vi "DataRootifier.vi"(4 "pathPlaceholder":string, 6 "replacePathPortion":string, 8 "mode":enum16{"Generalise", "Localise"}(ring)=enum."Localise", 11 "pathIn":path) -> (3 "pathOut":path)   [LabVIEW 2022 SP3]
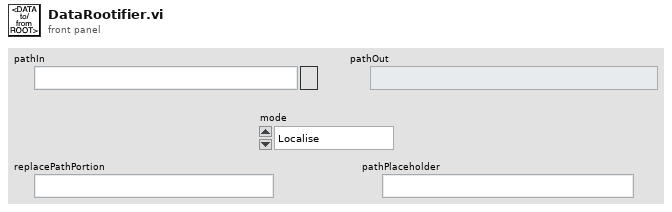
[diagram p1: front panel]
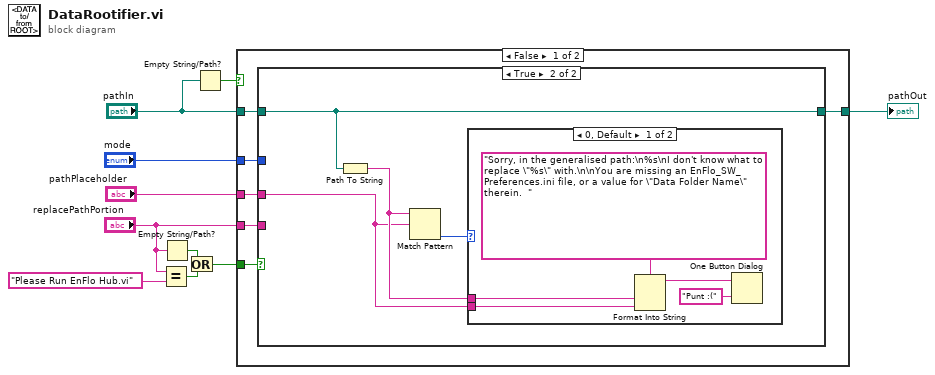
[diagram p0: block diagram]
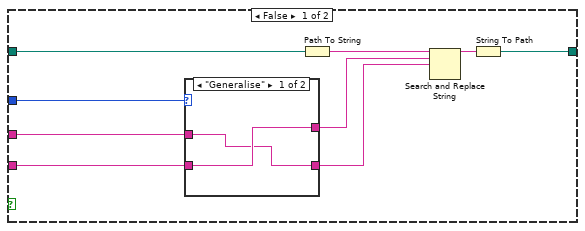
[diagram p2: hidden frame]
diagram:
  n1 = Equal?(x="replacePathPortion", y="Please Run EnFlo Hub.vi") -> (x = y?=w5:bool)
  n2 = Empty String/Path?(string/path="replacePathPortion") -> (empty?=w6:bool)
  n3 = Or(x=w6, y=w5) -> (x .or. y?=w7:bool)
  n4 = Empty String/Path?(string/path="pathIn") -> (empty?=w3:bool)
  n5 = case shown="False" w3 {
    tunnel: [w16 w39] -> w10
    tunnel: "pathIn" -> [w15 w39]
    tunnel: "replacePathPortion" -> [w14 _]
    tunnel: w7 -> [w13 _]
    tunnel: "pathPlaceholder" -> [w12 _]
    tunnel: "mode" -> [w11 _]
    frame False {
      n6 = case shown="True" w13 {
        tunnel: [w25 w33] -> w16
        tunnel: w15 -> [w22 w33]
        tunnel: w14 -> [w19 _]
        tunnel: w12 -> [w18 w30]
        tunnel: w11 -> [w17 _]
        frame False {
          n7 = case shown="\"Generalise\"" w17 {
            tunnel: [w27 w29] -> w21
            tunnel: w18 -> [w26 w29]
            tunnel: [w26 w28] -> w20
            tunnel: w19 -> [w27 w28]
            frame "Generalise" {
            }
            frame "Localise", Default {
            }
          }
          n8 = Path To String(path=w22) -> (string=w23:string)
          n9 = Search and Replace String(input string=w23, search string=w21, replace string=w20) -> (result string=w24:string)  [unwired: 5 in, 3 out]
          n10 = String To Path(string=w24) -> (path=w25:path)
        }
        frame True {
          n11 = Path To String(path=w33) -> (string=w31:string)
          n12 = Match Pattern(string=w31, regular expression=w30) -> (offset past match=w32:i32)  [unwired: 1 in, 3 out]
          n13 = case shown="0, Default" w32 {
            tunnel: w31 -> [w38 _]
            tunnel: w30 -> [w37 _]
            frame 0, Default {
              n14 = Format Into String(format string="Sorry, in the generalised path:\n%s\nI don't know what to replace \"%s\" with.\n\nYou are missing an EnFlo_SW_Preferences.ini file, or a value for \"Data Folder Name\" therein.  ", w38, w37) -> (resulting string=w35:string)  [unwired: 2 in, 1 out]
              n15 = One Button Dialog(message=w35, button name ("OK")="Punt :(") -> ()  [unwired: 1 out]
            }
            frame -1 {
            }
          }
        }
      }
    }
    frame True {
    }
  }
  "pathOut" <- w10
